vi "input.vi"(8 "error in":errorcluster, 10 "input data table in":T1, 11 "shared memory module":refnum<class "Shared Memory Runtime.lvclass">) -> (0 "error out":errorcluster, 2 "input data table out":T1, 3 "shared memory module out":refnum<class "Shared Memory Runtime.lvclass">)   [LabVIEW 2013, in "Shared Memory Runtime.lvclass"]
doc: "Provides an interface for reading data from a module at runtime. While this interface performs no operations, a child should provide an override which may read from any open sessions, references, or interfaces.Copyright 2016 National Instruments Corporation\n\nLicensed under the Apache License, Version 2.0 (the \"License\"); you may not use this file except in compliance with the License. You may obtain a copy of the License at http://www.apache.org/licenses/LICENSE-2.0\nUnless required by applicable law or agreed to in writing, software distributed under the License is distributed on an \"AS IS\" BASIS, WITHOUT WARRANTIES OR CONDITIONS OF ANY KIND, either express or implied. See the License for the specific language governing permissions and limitations under the License."
uses:
  Shared Memory Runtime.lvclass
  <vilib>/NI/Tag Bus/table/data table.ctl
  Shared Memory Runtime.lvclass/Shared Memory Runtime.ctl
  <vilib>/NI/Tag Bus/table/data polymorphs/write many/write Doubles.vi
  <vilib>/NI/Tag Bus/table/data table.lvlib
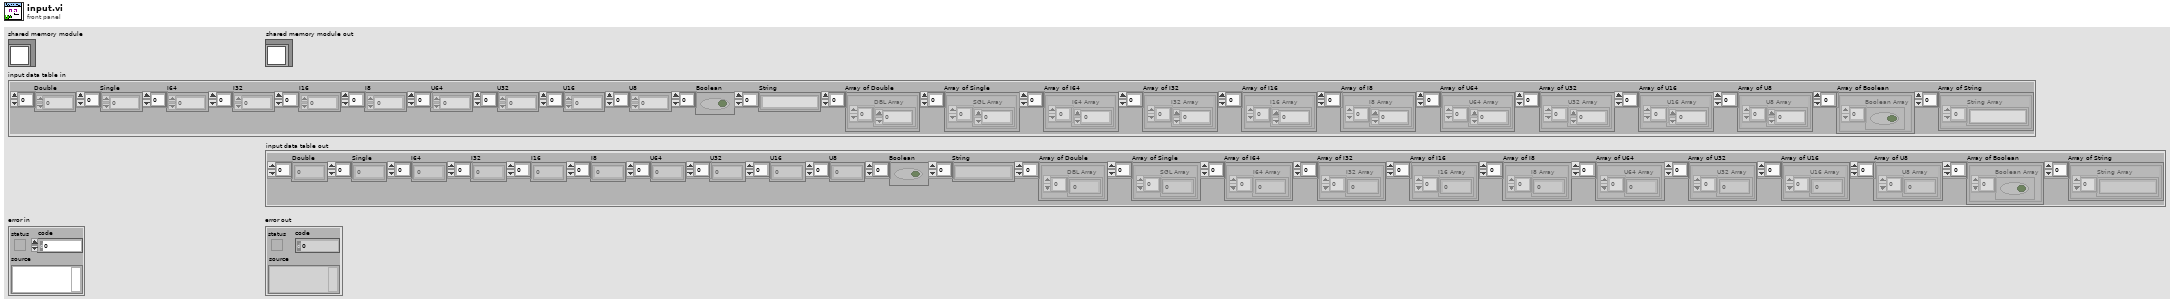
[diagram p1: front panel]
types:
  T1 = typedef "tag bus.lvlib/data table.lvlib/data table.ctl" = cluster{"Double":dbl[], "Single":sgl[], "I64":i64[], "I32":i32[], "I16":i16[], "I8":i8[], "U64":u64[], "U32":u32[], "U16":u16[], "U8":u8[], "Boolean":bool[], "String":string[], "Array of Double":cluster{"DBL Array":dbl[]}[], "Array of Single":cluster{"SGL Array":sgl[]}[], "Array of I64":cluster{"I64 Array":i64[]}[], "Array of I32":cluster{"I32 Array":i32[]}[], "Array of I16":cluster{"I16 Array":i16[]}[], "Array of I8":cluster{"I8 Array":i8[]}[], "Array of U64":cluster{"U64 Array":u64[]}[], "Array of U32":cluster{"U32 Array":u32[]}[], "Array of U16":cluster{"U16 Array":u16[]}[], "Array of U8":cluster{"U8 Array":u8[]}[], "Array of Boolean":cluster{"Boolean Array":bool[]}[], "Array of String":cluster{"String Array":string[]}[]}
  T2 = typedef "Shared Memory Runtime.lvclass/shared memory module runtime.ctl" = cluster{"refnum":refnum<file>, "name":string, "data type":T3, "number of tags":i32, "indices":cluster{"index":i32[]}, "data array":cluster{"data":dbl[]}, "file array":cluster{"data":dbl[]}}
  T3 = typedef "tag bus.lvlib/tag descriptor.lvclass/Data Type.ctl" = enum16{"Double", "Single", "I64", "I32", "I16", "I8", "U64", "U32", "U16", "U8", "Boolean", "String", "Array of Double", "Array of Single", "Array of I64", "Array of I32", "Array of I16", "Array of I8", "Array of U64", "Array of U32", "Array of U16", "Array of U8", "Array of Boolean", "Array of String"}
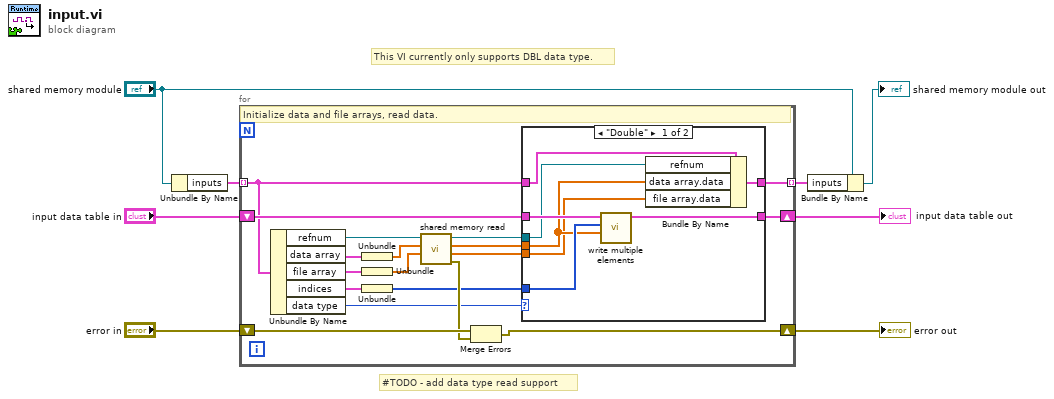
[diagram p0: block diagram]
diagram:
  # "#TODO - add data type read support"
  # "This VI currently only supports DBL data type."
  n1 = Unbundle By Name("shared memory module") -> ("inputs"=w4:T2[])
  n2 = for {
    tunnel: w4 -> [w12] mode=indexing
    shift-right: [w19] -> w5
    shift-left: "error in" -> [w21]
    shift-right: [w16] -> w8
    shift-left: "input data table in" -> [w15]
    tunnel: [w9] -> w2 mode=indexing
    # "Initialize data and file arrays, read data."
    n3 = Unbundle By Name(w12) -> ("refnum"=w26:refnum<file>, "data array"=w25:cluster{"data":dbl[]}, "file array"=w23:cluster{"data":dbl[]}, "indices"=w14:cluster{"index":i32[]}, "data type"=w13:T3)
    n4 = Unbundle(w25) -> ("data"=w24:dbl[])
    n5 = Unbundle(w23) -> ("data"=w22:dbl[])
    n6 = Unbundle(w14) -> ("index"=w18:i32[])
    n7 = call "shared memory read.vi"("file array"=w22, "data array"=w24, "refnum in"=w26) -> ("error out"=w20:errorcluster, "file array out"=w10:dbl[], "data array out"=w17:dbl[], "refnum out"=w11:refnum<file>)  [unwired: 4 in, 1 out]
    n8 = Merge Errors(w21, w20) -> (w19:errorcluster)
    n9 = case shown="\"Double\"" w13 {
      tunnel: w18 -> [w32 _]
      tunnel: w15 -> [w34 w36]
      tunnel: [w33 w36] -> w16
      tunnel: w17 -> [w29 _]
      tunnel: w12 -> [w31 w35]
      tunnel: w11 -> [w30 _]
      tunnel: w10 -> [w28 _]
      tunnel: [w27 w35] -> w9
      frame "Double" {
        n10 = call-poly <vilib>:"write multiple elements.vi"("values"=w29, "indices"=w32, "data table in"=w34) -> ("data table out"=w33:T1)  [unwired: 8 in]
        n11 = Bundle By Name(cluster=w31, "refnum"=w30, "data array.data"=w29, "file array.data"=w28) -> (w27:T2)
      }
      frame Default {
      }
    }
  }
  "error out" <- w5
  "input data table out" <- w8
  n12 = Bundle By Name(cluster="shared memory module", "inputs"=w2) -> (→"shared memory module out":refnum<class "Shared Memory Runtime.lvclass">)
